vi "CleanUp Diagram.vi"(8 "error in (no error)":errorcluster, 10 "Top Level Diagram":refnum<vi>, 11 "Initial Sequence in":refnum<class "Main Sequence.lvclass">) -> (0 "error out":errorcluster, 3 "Initial Sequence out":refnum<class "Main Sequence.lvclass">)   [LabVIEW 2025, in "Main Sequence.lvclass"]
uses:
  Main Sequence.lvclass
  Structures/Structures.lvclass/Structures.ctl
  Structures/Read Structure.vi
panel:
  out "Cluster":cluster{u32, u32}
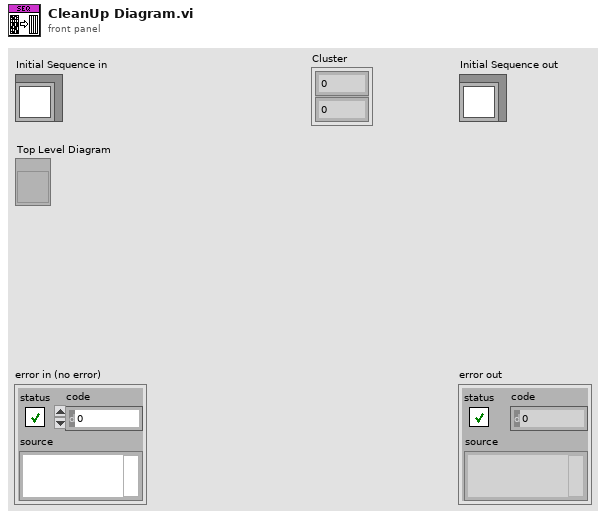
[diagram p1: front panel]
types:
  T1 = enum32{"Top Edges", "Vertical Centers", "Bottom Edges", "Vertical Gap", "Vertical Compress", "Left Edges", "Horizontal Centers", "Right Edges", "Horizontal Gap", "Horizontal Compress"}
  T2 = enum32{"Top Edges", "Vertical Centers", "Bottom Edges", "Left Edges", "Horizontal Centers", "Right Edges"}
  T3 = typedef "LVPositionTypeDef.ctl" = cluster{"Left":i32, "Top":i32}
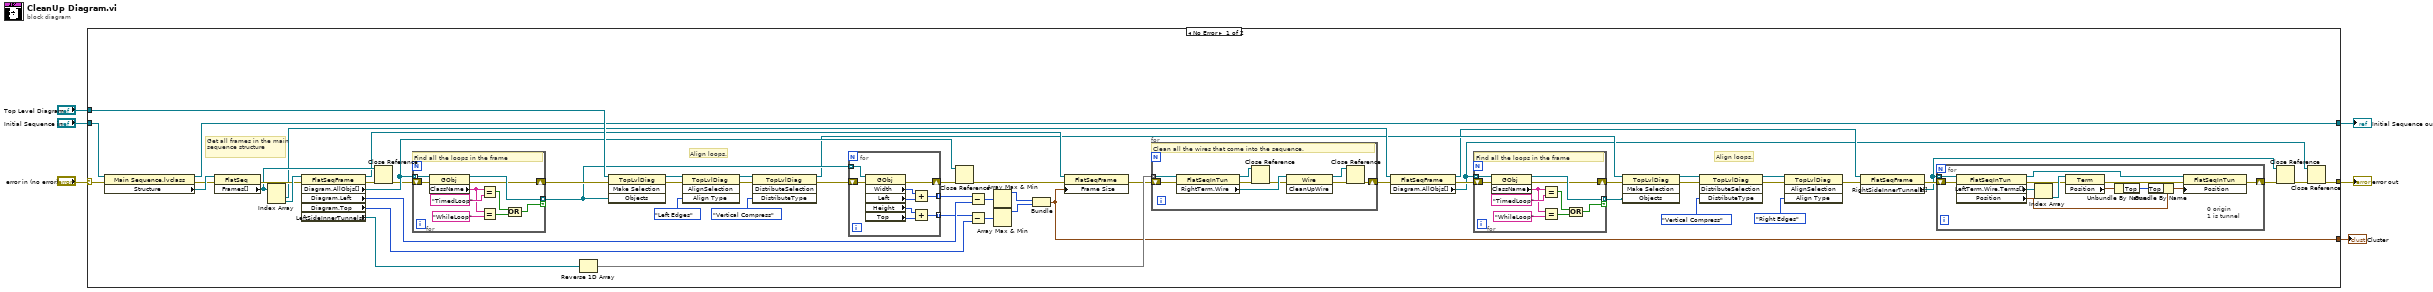
[diagram p0: block diagram]
diagram:
  n1 = case shown="No Error" "error in (no error)" {
    selector: "error in (no error)" -> [w52 w112]
    tunnel: "Initial Sequence in" -> [w53 w113]
    tunnel: "Top Level Diagram" -> [w51 _]
    tunnel: [w10 w112] -> w3
    tunnel: [w49 w113] -> w2
    tunnel: [w32 _] -> w1
    frame No Error {
      # "Align loops."
      # "Align loops."
      # "Get all frames in the main sequence structure"
      n2 = property class="Main Sequence.lvclass"(reference=w53, error in=w52) -> (reference out=w49:refnum<class "Main Sequence.lvclass">, error out=w60:errorcluster, "Structure"=w61:refnum<vi>)
      n3 = property class="FlatSeq"(reference=w61, error in=w60) -> (error out=w55:errorcluster, "Frames[]"=w44:refnum<vi>[])  [unwired: 1 out]
      n4 = Index Array(array=w44) -> (element #1=w30:refnum<vi>, element #2=w56:refnum<vi>)  [unwired: 2 in]
      n5 = property class="FlatSeqFrame"(reference=w56, error in=w55) -> (reference out=w31:refnum<vi>, error out=w46:errorcluster, "Diagram.AllObjs[]"=w47:refnum<vi>[], "Diagram.Left"=w41:i32, "Diagram.Top"=w40:i32, "LeftSideInnerTunnels[]"=w39:refnum<vi>[])
      n6 = Close Reference(reference=w44, error in (no error)=w46) -> (error out=w45:errorcluster)
      n7 = for {
        tunnel: w47 -> [w93] mode=indexing
        tunnel: [w88] -> w37 mode=indexing if=w84
        shift-right: [w86] -> w50
        shift-left: w45 -> [w87]
        # "Find all the loops in the frame"
        n8 = property class="GObj"(reference=w93, error in=w87) -> (reference out=w88:refnum<vi>, error out=w86:errorcluster, "ClassName"=w85:string)
        n9 = Equal?(x=w85, y="TimedLoop") -> (x = y?=w91:bool)
        n10 = Equal?(x=w85, y="WhileLoop") -> (x = y?=w89:bool)
        n11 = Compound Arithmetic op=OR(w91, w89) -> (w84:bool)
      }
      n12 = Reverse 1D Array(array=w39) -> (reversed array=w54:refnum<vi>[])
      n13 = invoke class="TopLvlDiag" method="Make Selection"(reference=w51, error in=w50, "Objects"=w37) -> (reference out=w59:refnum<vi>, error out=w58:errorcluster)  [unwired: 1 in, 2 out]
      n14 = invoke class="TopLvlDiag" method="AlignSelection"(reference=w59, error in=w58, "Align Type"=T2."Left Edges") -> (reference out=w19:refnum<vi>, error out=w18:errorcluster)  [unwired: 1 in, 2 out]
      n15 = invoke class="TopLvlDiag" method="DistributeSelection"(reference=w19, error in=w18, "DistributeType"=T1."Vertical Compress") -> (reference out=w16:refnum<vi>, error out=w17:errorcluster)  [unwired: 1 in, 2 out]
      n16 = for {
        tunnel: w37 -> [w102] mode=indexing
        shift-right: [w100] -> w38
        shift-left: w17 -> [w101]
        tunnel: [w97] -> w36 mode=indexing
        tunnel: [w94] -> w34 mode=indexing
        n17 = property class="GObj"(reference=w102, error in=w101) -> (error out=w100:errorcluster, "Width"=w98:u32, "Left"=w99:i32, "Height"=w96:u32, "Top"=w95:i32)  [unwired: 1 out]
        n18 = Add(x=w98, y=w99) -> (x+y=w97:u32)
        n19 = Add(x=w96, y=w95) -> (x+y=w94:u32)
      }
      n20 = Close Reference(reference=w47, error in (no error)=w38) -> (error out=w48:errorcluster)
      n21 = Subtract(x=w36, y=w41) -> (x-y=w35:u32[])
      n22 = Subtract(x=w34, y=w40) -> (x-y=w33:u32[])
      n23 = Array Max & Min(array=w35) -> (max value=w43:u32)  [unwired: 3 out]
      n24 = Array Max & Min(array=w33) -> (max value=w42:u32)  [unwired: 3 out]
      n25 = Bundle(w43, w42) -> (w32:cluster{u32, u32})  [unwired: 1 in]
      n26 = property class="FlatSeqFrame"(reference=w31, "Frame Size"=w32) -> ()  [unwired: 1 in, 2 out]
      n27 = for {
        tunnel: w54 -> [w111] mode=indexing
        shift-right: [w103] -> w29
        shift-left: w48 -> [w110]
        # "Clean all the wires that come into the sequence."
        n28 = property class="FlatSeqInTun"(reference=w111, error in=w110) -> (reference out=w107:refnum<vi>, error out=w108:errorcluster, "RightTerm.Wire"=w109:refnum<vi>)
        n29 = Close Reference(reference=w107, error in (no error)=w108) -> (error out=w106:errorcluster)
        n30 = invoke class="Wire" method="CleanUpWire"(reference=w109, error in=w106) -> (reference out=w104:refnum<vi>, error out=w105:errorcluster)  [unwired: 1 in, 1 out]
        n31 = Close Reference(reference=w104, error in (no error)=w105) -> (error out=w103:errorcluster)
      }
      n32 = property class="FlatSeqFrame"(reference=w30, error in=w29) -> (reference out=w13:refnum<vi>, error out=w28:errorcluster, "Diagram.AllObjs[]"=w7:refnum<vi>[])
      n33 = for {
        tunnel: w7 -> [w83] mode=indexing
        tunnel: [w78] -> w24 mode=indexing if=w74
        shift-right: [w76] -> w25
        shift-left: w28 -> [w77]
        # "Find all the loops in the frame"
        n34 = property class="GObj"(reference=w83, error in=w77) -> (reference out=w78:refnum<vi>, error out=w76:errorcluster, "ClassName"=w75:string)
        n35 = Equal?(x=w75, y="TimedLoop") -> (x = y?=w81:bool)
        n36 = Equal?(x=w75, y="WhileLoop") -> (x = y?=w79:bool)
        n37 = Compound Arithmetic op=OR(w81, w79) -> (w74:bool)
      }
      n38 = invoke class="TopLvlDiag" method="Make Selection"(reference=w16, error in=w25, "Objects"=w24) -> (reference out=w27:refnum<vi>, error out=w26:errorcluster)  [unwired: 1 in, 2 out]
      n39 = invoke class="TopLvlDiag" method="DistributeSelection"(reference=w27, error in=w26, "DistributeType"=T1."Vertical Compress") -> (reference out=w22:refnum<vi>, error out=w21:errorcluster)  [unwired: 1 in, 2 out]
      n40 = invoke class="TopLvlDiag" method="AlignSelection"(reference=w22, error in=w21, "Align Type"=T2."Right Edges") -> (error out=w14:errorcluster)  [unwired: 1 in, 3 out]
      n41 = property class="FlatSeqFrame"(reference=w13, error in=w14) -> (error out=w12:errorcluster, "RightSideInnerTunnels[]"=w8:refnum<vi>[])  [unwired: 1 out]
      n42 = for {
        tunnel: w8 -> [w73] mode=indexing
        shift-right: [w64] -> w9
        shift-left: w12 -> [w63]
        # "0 origin\n1 is tunnel"
        n43 = property class="FlatSeqInTun"(reference=w73, error in=w63) -> (reference out=w68:refnum<vi>, error out=w70:errorcluster, "LeftTerm.Wire.Terms[]"=w72:refnum<vi>[], "Position"=w62:T3)
        n44 = Index Array(array=w72) -> (element=w71:refnum<vi>)  [unwired: 1 in]
        n45 = property class="Term"(reference=w71, error in=w70) -> (error out=w65:errorcluster, "Position"=w69:T3)  [unwired: 1 out]
        n46 = Unbundle By Name(w69) -> ("Top"=w67:i32)
        n47 = Bundle By Name(cluster=w62, "Top"=w67) -> (w66:T3)
        n48 = property class="FlatSeqInTun"(reference=w68, error in=w65, "Position"=w66) -> (error out=w64:errorcluster)  [unwired: 1 out]
      }
      n49 = Close Reference(reference=w8, error in (no error)=w9) -> (error out=w11:errorcluster)
      n50 = Close Reference(reference=w7, error in (no error)=w11) -> (error out=w10:errorcluster)
    }
    frame Error {
    }
  }
  "error out" <- w3
  "Initial Sequence out" <- w2
  "Cluster" <- w1
